vi "ao_dc_voltage_pc_timed.vi"() -> ()   [LabVIEW 2020]
panel:
  in  "Stop":bool
  out "error out":errorcluster caption="错误输出"
  out "Voltage":sgl
  in  "Chan":u8
  in  "DevIndex":i32
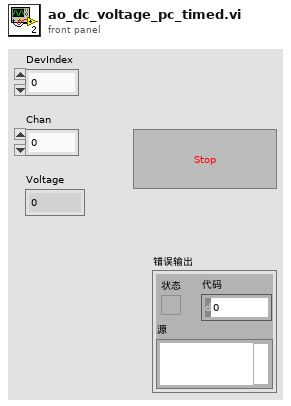
[diagram p1: front panel]
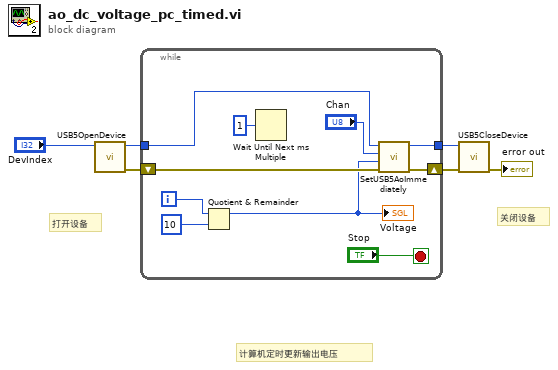
[diagram p0: block diagram]
diagram:
  # "关闭设备"
  # "计算机定时更新输出电压"
  # "打开设备"
  n1 = call "USB5OpenDevice.vi"("DevIndex"="DevIndex") -> ("error out"=w6:errorcluster, "DevIndex Out"=w4:i32)  [unwired: 9 in]
  n2 = while {
    shift-right: [w12] -> w1
    shift-left: w6 -> [w14]
    tunnel: w4 -> [w16]
    tunnel: [w13] -> w2
    i -> [w10]
    stop <- "Stop" stop-if-true
    n3 = Quotient & Remainder(x=w10, y=10) -> (x-y*floor(x/y)=w8:i32)  [unwired: 1 out]
    "Voltage" <- w8
    n4 = Wait Until Next ms Multiple(millisecond multiple=u32 1 ("毫秒倍数")) -> ()  [unwired: 1 out]
    n5 = call "SetUSB5AoImmediately.vi"("错误输入（无错误）"=w14, "Voltage"=w8, "Chan"="Chan", "DevIndex"=w16) -> ("错误输出"=w12:errorcluster, "DevIndex Out"=w13:i32)  [unwired: 6 in]
  }
  n6 = call "USB5CloseDevice.vi"("错误输入（无错误）"=w1, "DevIndex"=w2) -> ("error out"=→"error out":errorcluster)  [unwired: 8 in, 1 out]
